vi "cause_memory_leak.vi"() -> ()   [LabVIEW 2020]
uses:
  <vilib>/Rock Robotics/WPI/ThirdParty/JAS_Junk/TrajLib/Trajectory_Library.lvlib
  Subsystems/Swerve/swerve_globals.vi
panel:
  in  "Cause Memory Leak?":bool
  out "y":cluster{"Y":dbl, "Y":dbl}(graph)
  out "x":cluster{"X":dbl, "X":dbl}(graph)
  out "Robot Position":T1(graph)
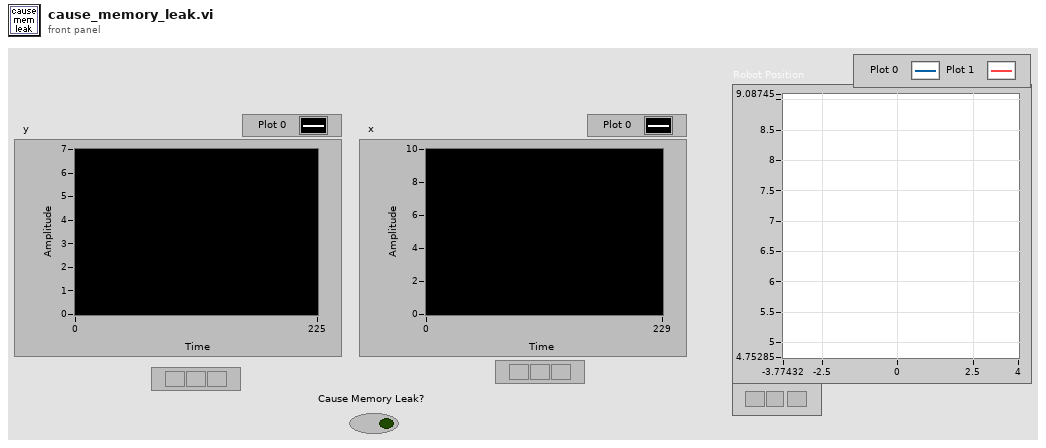
[diagram p1: front panel]
types:
  T1 = cluster{"output array":dbl[], "output array":dbl[]}[]
  T2 = typedef "Trajectory_Library.lvlib/POSE2D.ctl" = cluster{"TRANSLATION":T3, "ROTATION":T4}
  T3 = typedef "Trajectory_Library.lvlib/TRANSLATION2D.ctl" = cluster{"X":dbl, "Y":dbl}
  T4 = typedef "Trajectory_Library.lvlib/ROTATION2D.ctl" = cluster{"VALUE":dbl, "COS":dbl, "SIN":dbl}
  T5 = cluster{"output array":dbl[], "output array":dbl[]}
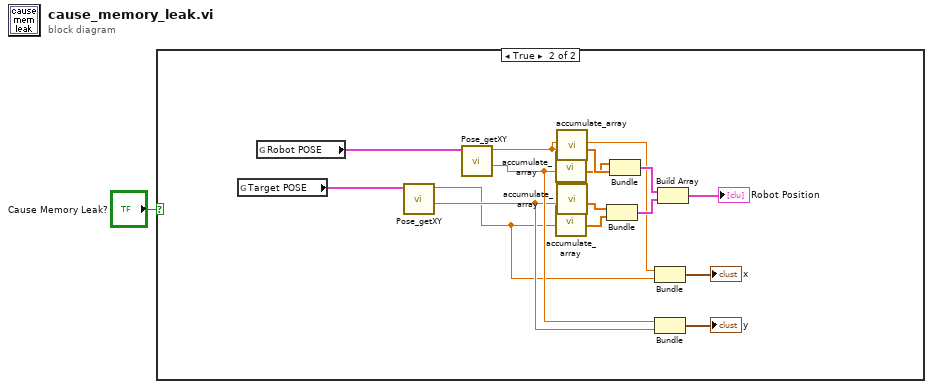
[diagram p0: block diagram]
diagram:
  n1 = case shown="True" "Cause Memory Leak?" {
    frame False {
      # "no?\nwhy not?\n:("
    }
    frame True {
      n2 = global read "swerve_globals.vi" "Target POSE"() -> (w9:T2)
      n3 = global read "swerve_globals.vi" "Robot POSE"() -> (w2:T2)
      n4 = call <vilib>:"Pose_getXY.vi"("in POSE"=w9) -> ("Y"=w6:dbl, "X"=w5:dbl)  [unwired: 9 in]
      n5 = call <vilib>:"Pose_getXY.vi"("in POSE"=w2) -> ("Y"=w7:dbl, "X"=w8:dbl)  [unwired: 9 in]
      n6 = call "accumulate_array.vi"("value"=w7) -> ("output array"=w15:dbl[])  [unwired: 10 in]
      n7 = call "accumulate_array.vi"("value"=w5) -> ("output array"=w13:dbl[])  [unwired: 10 in]
      n8 = call "accumulate_array.vi"("value"=w8) -> ("output array"=w16:dbl[])  [unwired: 10 in]
      n9 = call "accumulate_array.vi"("value"=w6) -> ("output array"=w14:dbl[])  [unwired: 10 in]
      n10 = Bundle("output array"=w14, "output array"=w13) -> (w11:T5)  [unwired: 1 in]
      n11 = Bundle("output array"=w15, "output array"=w16) -> (w12:T5)  [unwired: 1 in]
      n12 = Bundle("X"=w8, "X"=w5) -> (→"x":cluster{"X":dbl, "X":dbl})  [unwired: 1 in]
      n13 = Bundle("Y"=w7, "Y"=w6) -> (→"y":cluster{"Y":dbl, "Y":dbl})  [unwired: 1 in]
      n14 = Build Array(w12, w11) -> (→"Robot Position":T1)
    }
  }
